vi "is_done.vi"(8 "error in (no error)":errorcluster, 11 "Analog_Output in":refnum<class "Analog_Output.lvclass">) -> (0 "error out":errorcluster, 2 "task done?":bool, 3 "Analog_Output out":refnum<class "Analog_Output.lvclass">)   [LabVIEW 2013, in "Analog_Output.lvclass"]
uses:
  Analog_Output.lvclass
  Analog_Output.lvclass/Analog_Output.ctl
  Globals.vi
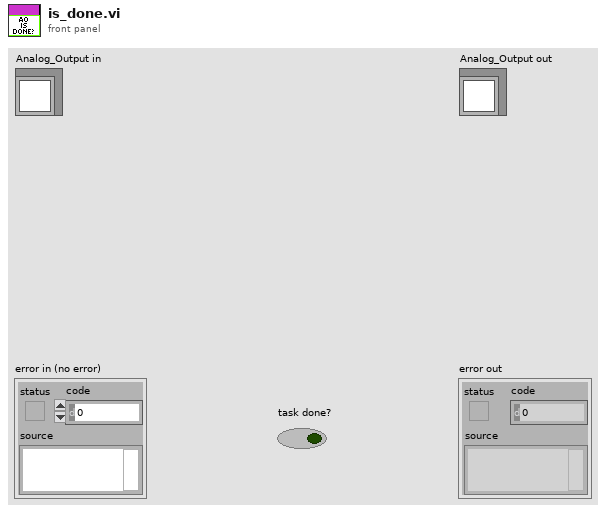
[diagram p1: front panel]
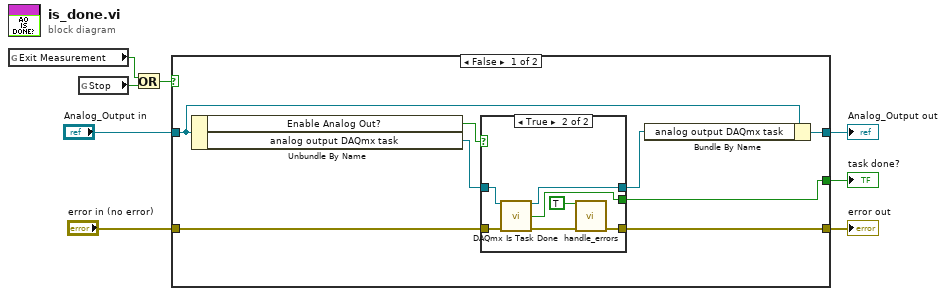
[diagram p0: block diagram]
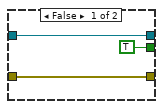
[diagram p2: hidden frame]
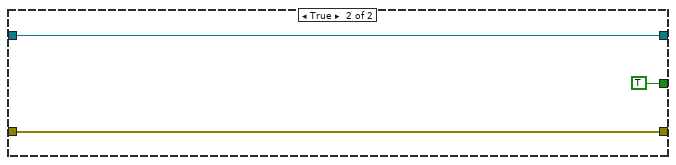
[diagram p3: hidden frame]
diagram:
  n1 = global read "Globals.vi" "Exit Measurement"() -> (w5:bool)
  n2 = global read "Globals.vi" "Stop"() -> (w4:bool)
  n3 = Or(x=w5, y=w4) -> (x .or. y?=w3:bool)
  n4 = case shown="False" w3 {
    tunnel: [w15 w28] -> w6
    tunnel: [w12 w29] -> w7
    tunnel: "Analog_Output in" -> [w13 w29]
    tunnel: "error in (no error)" -> [w10 w28]
    tunnel: [w9 TRUE ("Exit Measurement")] -> w1
    frame False {
      n5 = Unbundle By Name(w13) -> ("Enable Analog Out?"=w16:bool, "analog output DAQmx task"=w14:refnum<k21>)
      n6 = case shown="True" w16 {
        tunnel: w10 -> [w19 w26]
        tunnel: [w19 w21] -> w15
        tunnel: w14 -> [w18 w25]
        tunnel: [w18 w24] -> w11
        tunnel: [TRUE ("task done?") w23] -> w9
        frame False {
        }
        frame True {
          n7 = call <vilib>:"DAQmx Is Task Done.vi"("task/channels in"=w25, "error in"=w26) -> ("task out"=w24:refnum<k21>, "task done?"=w23:bool, "error out"=w22:errorcluster)  [unwired: 11 in]
          n8 = call "handle_errors.vi"("Exit Operation"=TRUE ("Exit Measurement"), "error in (no error)"=w22) -> ("error out"=w21:errorcluster)  [unwired: 13 in]
        }
      }
      n9 = Bundle By Name(cluster=w13, "analog output DAQmx task"=w11) -> (w12:refnum<class "Analog_Output.lvclass">)
    }
    frame True {
    }
  }
  "error out" <- w6
  "Analog_Output out" <- w7
  "task done?" <- w1
